vi "Set Mode.vi"(7 "Ref Mode":refnum<vi>, 8 "error in":errorcluster, 9 "Head Channel":i16, 10 "Pulsar Handle":i16, 11 "OphirFastX (in)":refnum<k7>) -> (0 "error out":errorcluster, 3 "OphirFastX (out)":refnum<k7>)   [LabVIEW 2009]
panel:
  # "Guillaume Plateau - yguig2@yahoo.fr"
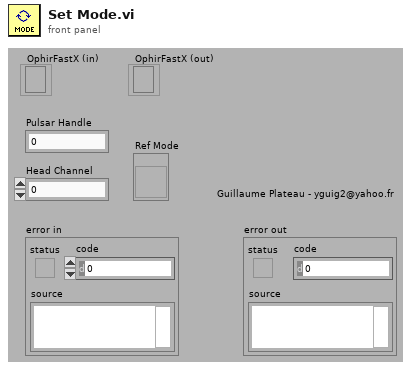
[diagram p1: front panel]
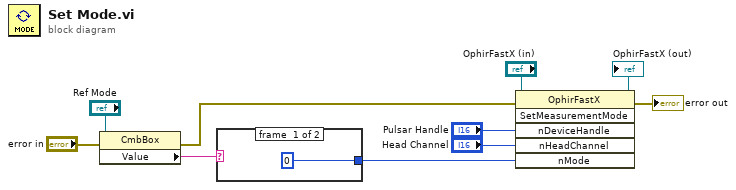
[diagram p0: block diagram]
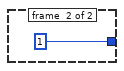
[diagram p2: hidden frame]
diagram:
  n1 = property class="CmbBox"(reference="Ref Mode", error in="error in") -> (error out=w1:errorcluster, "Value"=w4:string)  [unwired: 1 out]
  n2 = case shown="\"Energy\", Default" w4 {
    tunnel: [i16 0 ("nMode") i16 1 ("nMode")] -> w3
    frame #0 {
    }
    frame #1 {
    }
  }
  n3 = invoke class="OphirFastX" method="SetMeasurementMode"(reference="OphirFastX (in)", error in=w1, "nDeviceHandle"="Pulsar Handle", "nHeadChannel"="Head Channel", "nMode"=w3) -> (reference out=→"OphirFastX (out)":refnum<k7>, error out=→"error out":errorcluster)  [unwired: 1 in, 4 out]
